vi "Deploy-ExtractImage.vi"(8 "error in (no error)":errorcluster, 11 "Selected Image File":path) -> (0 "error out":errorcluster, 3 "AppImage Properties":T1)   [LabVIEW 2021]
uses:
  TypeDefs/AppImageProperties.ctl
  TypeDefs/FPGA_Properties_Element.ctl
  <vilib>/Utility/sysdir.llb/System Directory Type.ctl
  95eed4b0-98c6-4b89-a3fd-57541fbdea9d.vi
  <userlib>/_OpenG.lib/lvzip/lvzip.llb/subVI/ZLIB Extract All Files To Dir (Path)__ogtk.vi
  <vilib>/JDP Science/JSONtext/JSON text to Variant.vi
  <vilib>/JDP Science/JSONtext/LVClass Serializer/JSONtext LVClass Serializer.lvclass
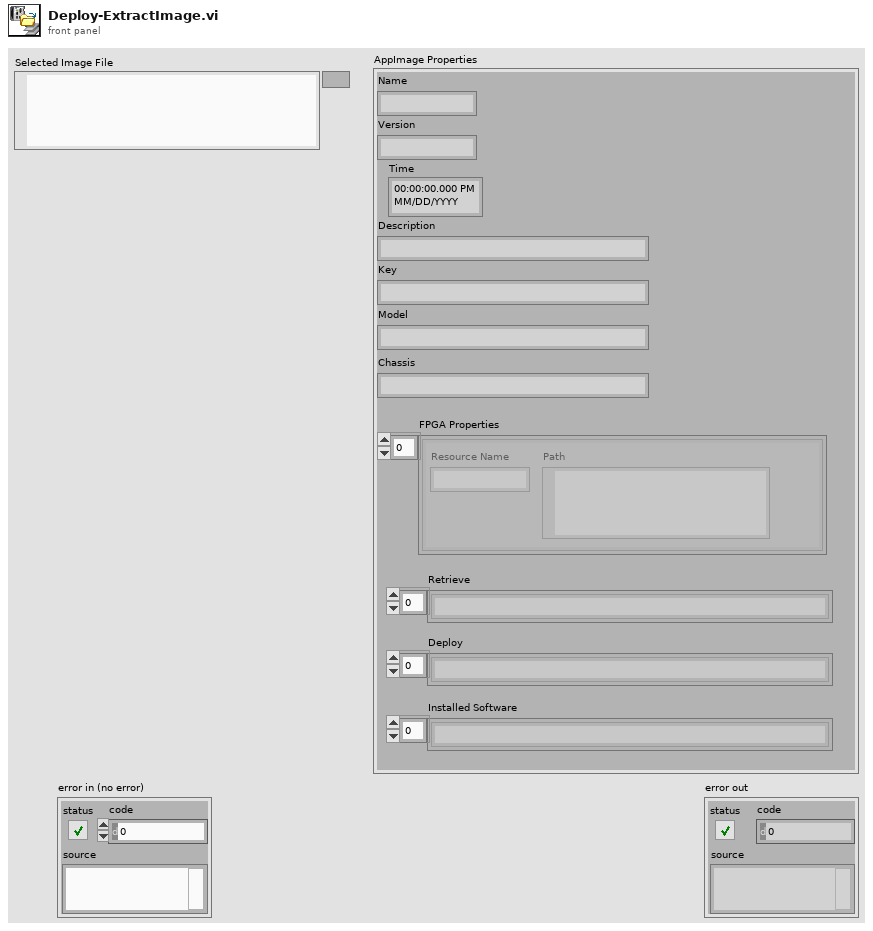
[diagram p1: front panel]
types:
  T1 = typedef "AppImageProperties.ctl" = cluster{"Name":string, "Version":string, "Time":timestamp, "Description":string, "Key":string, "Chassis":string, "FPGA Properties":T2[], "Model":string, "Retrieve":string[], "Deploy":string[], "Installed Software":string[]}
  T2 = typedef "FPGA_Properties_Element.ctl" = cluster{"Resource Name":string, "Path":path}
  T3 = typedef "System Directory Type.ctl" = i32
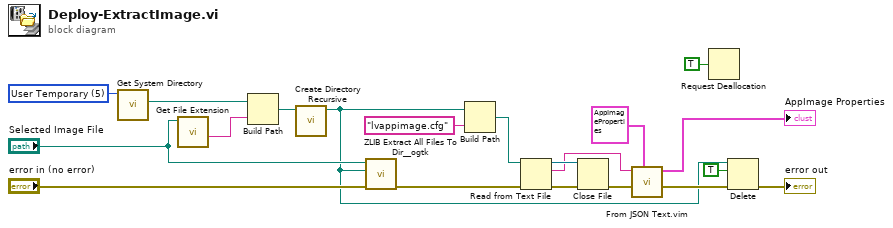
[diagram p0: block diagram]
diagram:
  w20 = T3 5 items=["User Home"=0, "User Desktop"=1, "User Documents"=2, "User Application Data"=3, "User Preferences"=4, "User Temporary"=5, "Public Documents"=6, "Public Application Data"=7, "Public Preferences"=8, "Public Cache"=13, "System Core Libraries"=9, "System Installed Libraries"=10, "Application Files"=11, "Boot Volume Root"=12] ("system directory type")
  n1 = call <vilib>:"Get System Directory.vi"("system directory type"=w20) -> ("system directory"=w19:path)  [unwired: 10 in]
  n2 = call <vilib>:"Get File Extension.vi"("file"="Selected Image File") -> ("filename without extension"=w16:string)  [unwired: 6 in, 4 out]
  n3 = Build Path(base path=w19, name or relative path=w16) -> (appended path=w17:path)
  n4 = call <vilib>:"Create Directory Recursive.vi"("directory"=w17) -> ("directory copy"=w2:path)  [unwired: 4 in, 2 out]
  n5 = call-poly <userlib>:"ZLIB Extract All Files To Dir__ogtk.vi"("error in (no error)"="error in (no error)", "destination directory (archive name without ending)"=w2, "archive name (file dialog)"="Selected Image File") -> ("error out"=w12:errorcluster)  [unwired: 6 in, 2 out]
  n6 = Build Path(base path=w2, name or relative path="lvappimage.cfg") -> (appended path=w13:path)
  n7 = Read from Text File(file (use dialog)=w13, error in=w12) -> (refnum out=w11:refnum<file>, text=w8:string, error out=w10:errorcluster)  [unwired: 2 in, 1 out]
  n8 = Close File(refnum=w11, error in=w10) -> (error out=w7:errorcluster)  [unwired: 1 out]
  n9 = call "From JSON Text.vim"("Data Type and Default Value"=T1 {"Name"="", "Version"="", "Time"=timestamp(0 s since 1904-01-01), "Description"="", "Key"="", "Chassis"="", "FPGA Properties"=[], "Model"="", "Retrieve"=[], "Deploy"=[], "Installed Software"=[]} ("AppImage Properties"), "error in (no error)"=w7, "JSON"=w8) -> ("error out"=w4:errorcluster, "Data out"=→"AppImage Properties":T1)  [unwired: 7 in]
  n10 = Request Deallocation(TRUE ("flag")) -> ()
  n11 = Delete(path (use dialog)=w2, entire hierarchy (F)=TRUE, error in=w4) -> (error out=→"error out":errorcluster)  [unwired: 2 in, 2 out]
